vi "Set All Component Settings.vi"(8 "error in (no error)":errorcluster, 10 "component settings":T1[](array[typedef]), 11 "Runtime Configuration in":refnum<class "Core Configuration.lvclass">) -> (0 "error out":errorcluster, 3 "Runtime Configuration out":refnum<class "Core Configuration.lvclass">)   [LabVIEW 2020, in "DSF Core.lvlib" / "Core Configuration.lvclass"]
uses:
  Core Configuration.lvclass
  Typedefs/DSF Settings Info.ctl
  Core Configuration.lvclass/Core Configuration.ctl
  DSF Core.lvlib
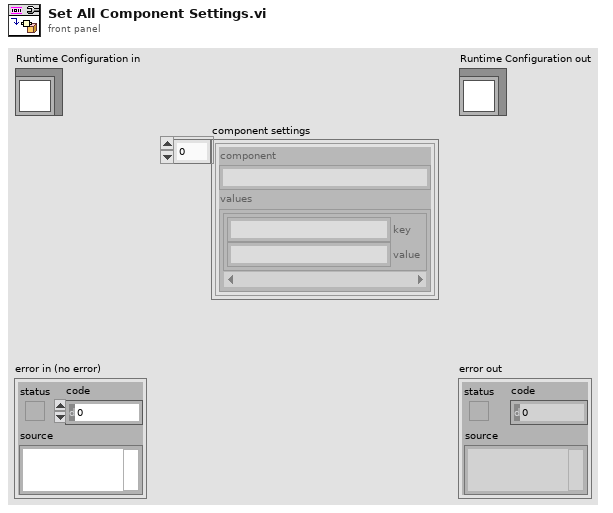
[diagram p1: front panel]
types:
  T1 = typedef "DSF Core.lvlib/DSF Settings Info.ctl" = cluster{"component":string, "values":cluster{"key":string, "value":string}[]}
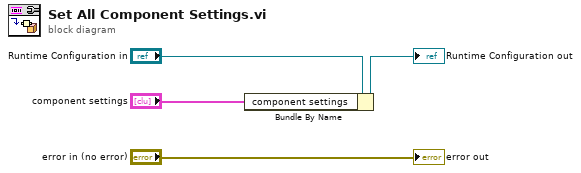
[diagram p0: block diagram]
diagram:
  n1 = Bundle By Name(cluster="Runtime Configuration in", "component settings"="component settings") -> (→"Runtime Configuration out":refnum<class "Core Configuration.lvclass">)
  "error out" <- "error in (no error)"
